vi "Degrees per second to degrees.vi"(7 "Initialize":bool, 10 "Sample time (ms)":u32, 11 "Rate of turn (°/s)":dbl) -> (3 "Degrees":dbl)   [LabVIEW 2011]
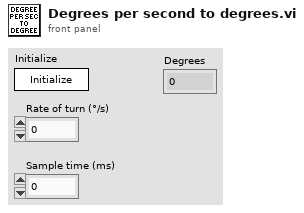
[diagram p1: front panel]
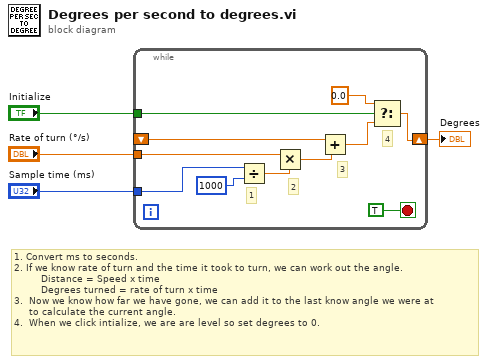
[diagram p0: block diagram]
diagram:
  # "1. Convert ms to seconds.\n2. If we know rate of turn and the time it took to turn, we can work out the angle.\n         Distance = Speed x time \n         Degrees turned = rate of turn x time\n3.  Now we know how far we have gone, we can add it to the last know angle we were at\n     to calculate the current angle.\n4.  When we click intialize, we are are level so set degrees to 0."
  n1 = while {
    tunnel: "Sample time (ms)" -> [w13]
    tunnel: "Rate of turn (°/s)" -> [w12]
    shift-right: [w7] -> w4
    shift-left: _ -> [w11]
    tunnel: "Initialize" -> [w9]
    stop <- TRUE stop-if-true
    # "4"
    # "3"
    # "2"
    # "1"
    n2 = Divide(x=w13, y=u32 1000) -> (x/y=w15:dbl)
    n3 = Multiply(x=w12, y=w15) -> (x*y=w5:dbl)
    n4 = Add(x=w11, y=w5) -> (x+y=w8:dbl)
    n5 = Select(t=0.0, s=w9, f=w8) -> (s? t:f=w7:dbl)
  }
  "Degrees" <- w4
